vi "探头窗口-12-网络版.vi"() -> ()   [LabVIEW 2017]
panel:
  in  "外部停止命令？":bool=TRUE
  out "引用-监测模式？":refnum<vi>
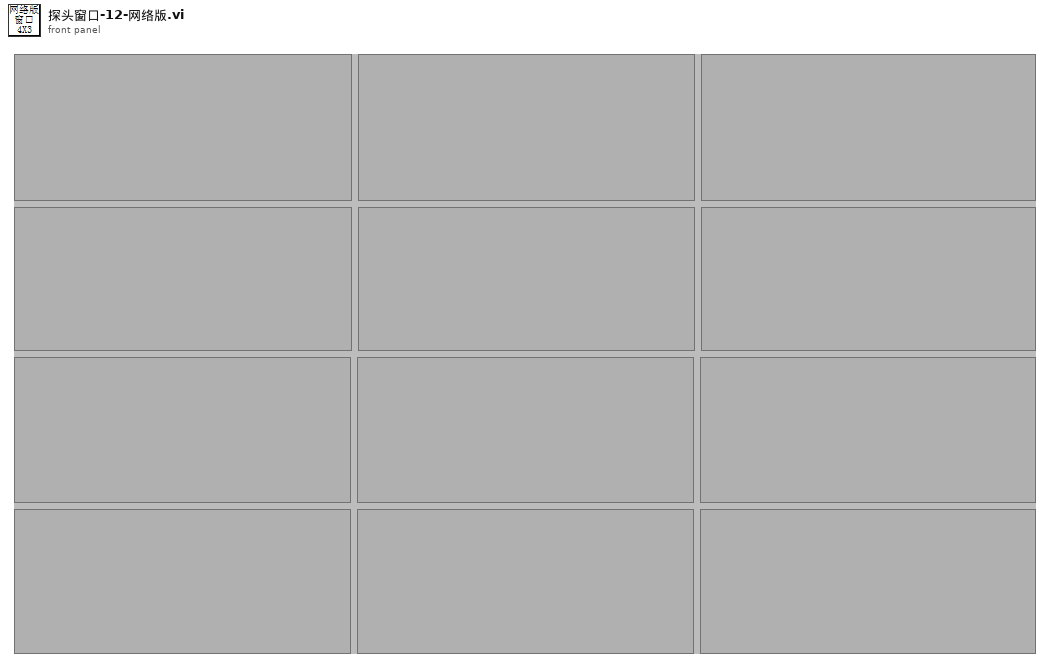
[diagram p1: front panel]
types:
  T1 = typedef "eventvkey.ctl" = enum16{"ASCII", "Enter", "Return", "Shift", "Ctrl", "Alt", "Cmd", "Opt", "Caps", "NumLock", "Clear", "Break", "Up", "Down", "Left", "Right", "Insert", "Delete", "Home", "End", "PageUp", "PageDown", "Escape", "Help", "Pause", "ScrollLock", "F1", "F2", "F3", "F4", "F5", "F6", "F7", "F8", "F9", "F10", "F11", "F12", "F13", "F14", "F15", "F16", "F17", "F18", "F19", "F20", "F21", "F22", "F23", "F24", "Play", "VolumeUp", "VolumeDown", "Mute", "Two Byte Char"}
  T2 = typedef "探头属性.ctl" = cluster{"探头地址与信息":T3, "测量值":T6, "限值":T7, "探头状态":T8, "累积记录":T9, "报警方式":T10}
  T3 = typedef "探测器信息.ctl" = cluster{"网络地址":string, "名称":string, "备注":string, "累积剂量":dbl, "累积限值":dbl, "硬件剂量率限值":T4, "剂量率限值1":dbl, "剂量率限值2":dbl, "报警方式":T5}
  T4 = typedef "探头剂量率限值选择.ctl" = enum16{"一级限值", "二级限值"}
  T5 = typedef "报警方式选择.ctl" = enum16{"常报警", "自动静音", "手动静音"}
  T6 = typedef "测量值.ctl" = cluster{"时间":timestamp, "数值":dbl}
  T7 = typedef "剂量率限值.ctl" = cluster{"限值1":dbl, "限值2":dbl, "探头限值":T4}
  T8 = typedef "探头状态.ctl" = enum16{"正常", "离线", "禁用", "一级报警", "二级报警", "累积报警"}
  T9 = typedef "单条累积记录.ctl" = cluster{"起始时间":timestamp, "结束时间":timestamp, "累积剂量":dbl}
  T10 = typedef "报警方式.ctl" = cluster{"报警方式":T5, "延迟计时":u16, "报警中？":bool}
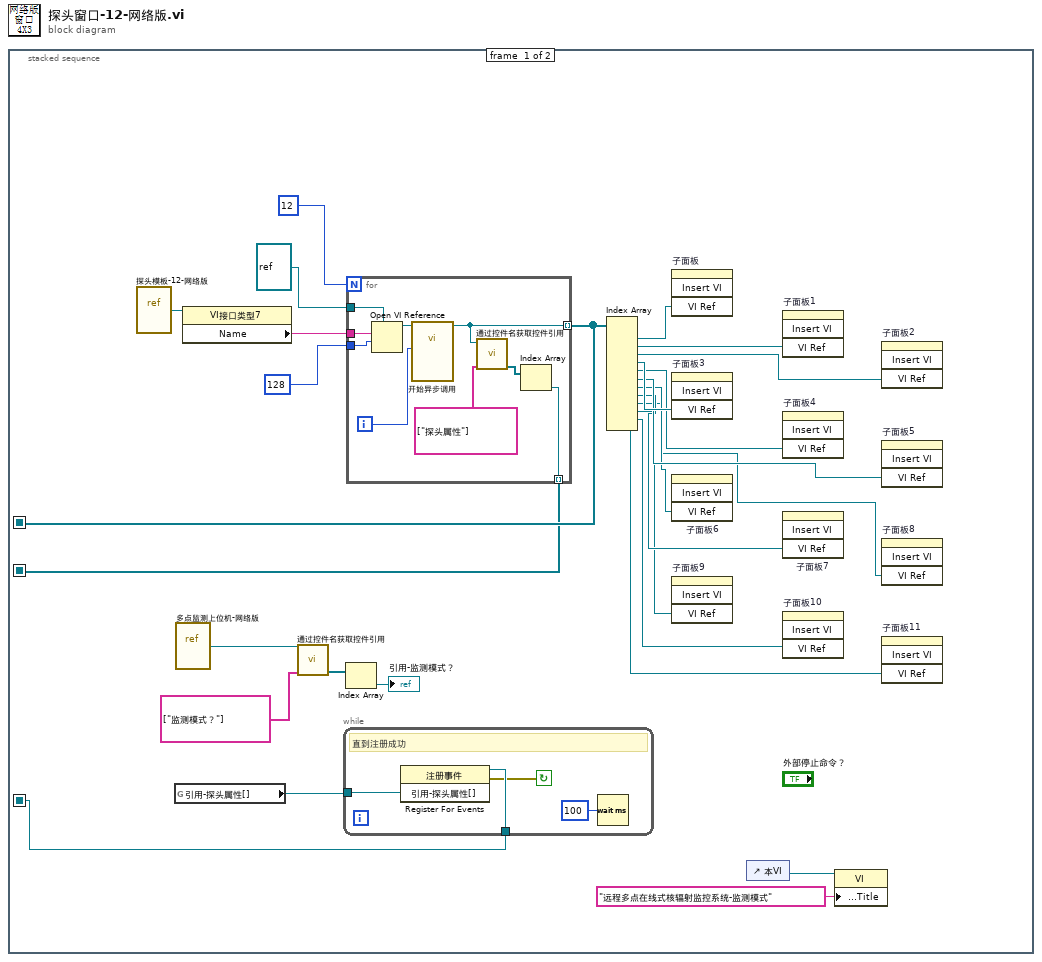
[diagram p0: block diagram]
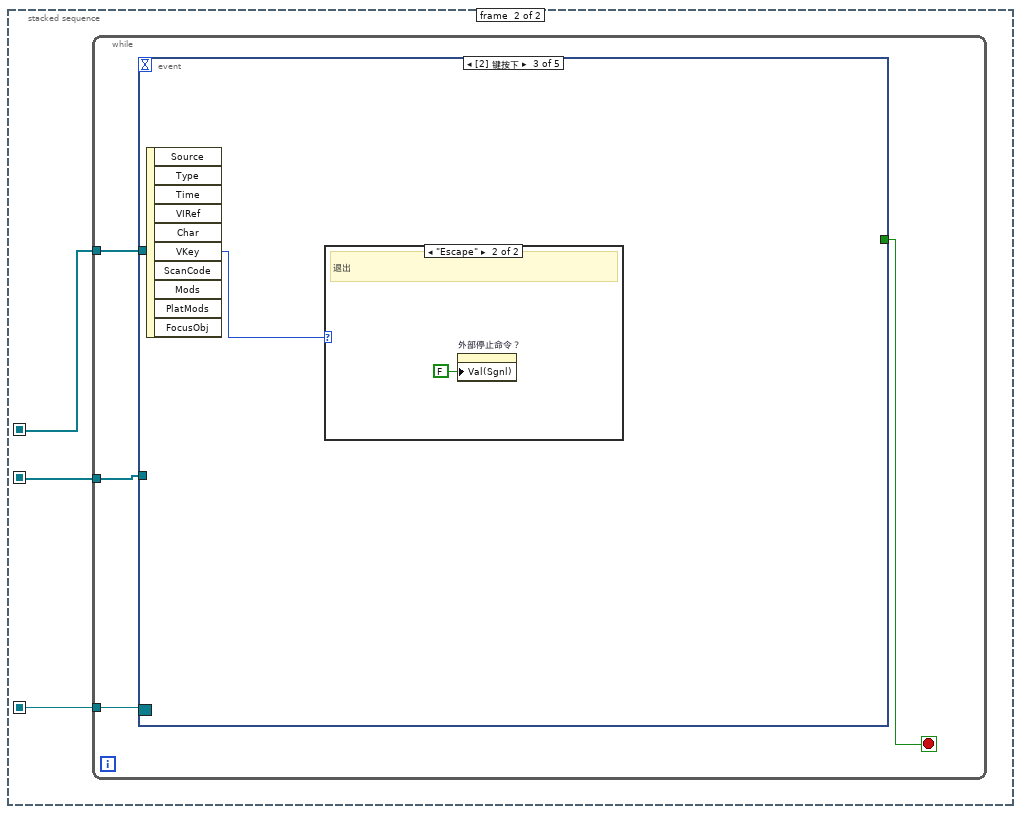
[diagram p2: hidden frame]
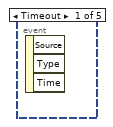
[diagram p3: hidden frame]
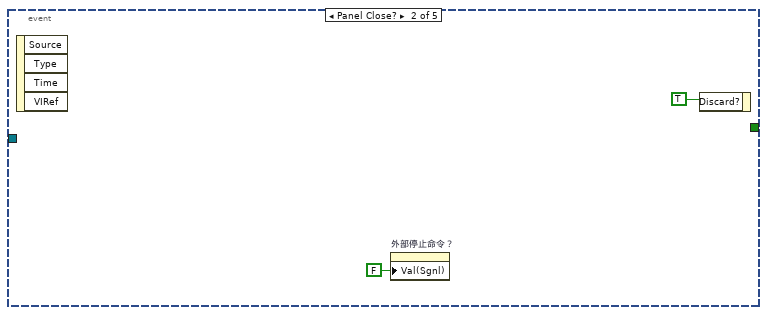
[diagram p4: hidden frame]
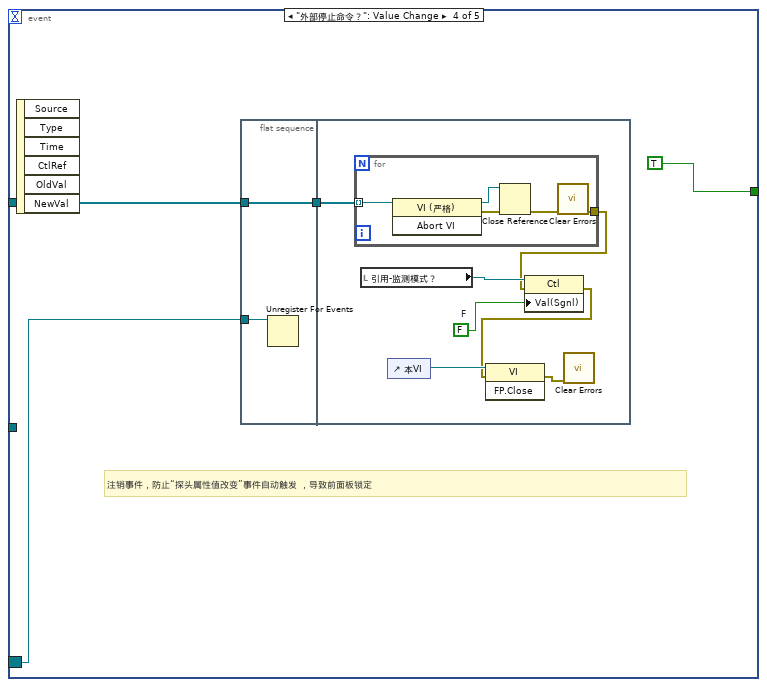
[diagram p6: hidden frame]
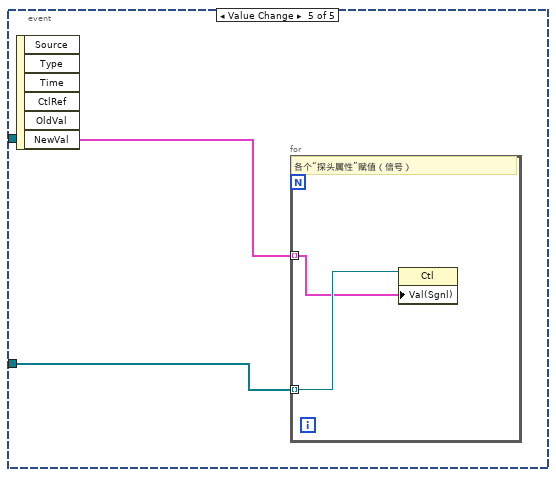
[diagram p7: hidden frame]
diagram:
  n1 = stacked-sequence {
    seq-local: [w23 _] -> [_ w43]
    seq-local: [w21 _] -> [_ w42]
    seq-local: [w1 _] -> [_ w41]
    frame #0 {
      n2 = vi-ref "探头模板-12-网络版.vi"() -> (w27:refnum<vi>)
      n3 = global read "全局变量-35点监测.vi" "引用-探头属性[]"() -> (w2:refnum<vi>)
      n4 = vi-ref "多点监测上位机-网络版.vi"() -> (w5:refnum<vi>)
      n5 = property class="VI接口类型7"(reference=w27) -> ("Name"=w26:string)  [unwired: 1 in, 2 out]
      n6 = call "通过控件名获取控件引用.vi"("控件名数组"=string[] ["监测模式？"], "VI引用"=w5) -> ("控件引用输出"=w7:refnum<vi>[])  [unwired: 7 in, 2 out]
      n7 = while {
        tunnel: w2 -> [w31]
        tunnel: [w30] -> w1
        stop <- w29 continue-if-true
        # "直到注册成功"
        n8 = register-events(w31) -> (reference out=w30:refnum<event-registration>, error out=w29:errorcluster)  [unwired: 2 in]
        n9 = Wait (ms)(milliseconds to wait=u32 100 ("等待时间（毫秒）")) -> ()  [unwired: 1 out]
      }
      n10 = Index Array(array=w7) -> (element=→"引用-监测模式？":refnum<vi>)  [unwired: 1 in]
      n11 = for "For循环" {
        N: 12 -> [_]
        tunnel: w26 -> [w40]
        tunnel: 128 ("选项") -> [w39]
        tunnel: refnum<vi> refnum ("类型说明符VI引用句柄（仅用于类型）") -> [w38]
        tunnel: [w33] -> w23 mode=indexing
        tunnel: [w34] -> w21 mode=indexing
        i -> [w32]
        n12 = Open VI Reference(type specifier VI Refnum (for type only)=w38, vi path=w40, options=w39) -> (vi reference=w35:refnum<vi>)  [unwired: 3 in, 1 out]
        n13 = call-by-ref "开始异步调用"(reference=w35, "探头序号"=w32) -> (reference out=w33:refnum<vi>)  [unwired: 12 in, 1 out]
        n14 = call "通过控件名获取控件引用.vi"("控件名数组"=string[] ["探头属性"], "VI引用"=w33) -> ("控件引用输出"=w37:refnum<vi>[])  [unwired: 7 in, 2 out]
        n15 = Index Array(array=w37) -> (element=w34:refnum<vi>)  [unwired: 1 in]
      }
      n16 = Index Array(array=w23) -> (element #1=w20:refnum<vi>, element #2=w19:refnum<vi>, element #3=w18:refnum<vi>, element #4=w17:refnum<vi>, element #5=w16:refnum<vi>, element #6=w15:refnum<vi>, element #7=w14:refnum<vi>, element #8=w13:refnum<vi>, element #9=w12:refnum<vi>, element #10=w11:refnum<vi>, element #11=w10:refnum<vi>, element #12=w9:refnum<vi>)  [unwired: 12 in]
      n17 = invoke on="子面板" class="子面板" method="Insert VI"("VI Ref"=w20) -> ()  [unwired: 3 in, 4 out]
      n18 = invoke on="子面板3" class="SubPnl" method="Insert VI"("VI Ref"=w17) -> ()  [unwired: 3 in, 4 out]
      n19 = invoke on="子面板6" class="SubPnl" method="Insert VI"("VI Ref"=w14) -> ()  [unwired: 3 in, 4 out]
      n20 = invoke on="子面板9" class="SubPnl" method="Insert VI"("VI Ref"=w11) -> ()  [unwired: 3 in, 4 out]
      n21 = control-ref of="本VI"() -> (w4:refnum<vi>)
      n22 = invoke on="子面板1" class="SubPnl" method="Insert VI"("VI Ref"=w19) -> ()  [unwired: 3 in, 4 out]
      n23 = invoke on="子面板4" class="SubPnl" method="Insert VI"("VI Ref"=w16) -> ()  [unwired: 3 in, 4 out]
      n24 = invoke on="子面板7" class="SubPnl" method="Insert VI"("VI Ref"=w13) -> ()  [unwired: 3 in, 4 out]
      n25 = invoke on="子面板10" class="SubPnl" method="Insert VI"("VI Ref"=w10) -> ()  [unwired: 3 in, 4 out]
      n26 = property class="VI"(reference=w4, "Front Panel.Title"="远程多点在线式核辐射监控系统-监测模式" ("前面板窗口:标题")) -> ()  [unwired: 1 in, 2 out]
      n27 = invoke on="子面板2" class="SubPnl" method="Insert VI"("VI Ref"=w18) -> ()  [unwired: 3 in, 4 out]
      n28 = invoke on="子面板5" class="SubPnl" method="Insert VI"("VI Ref"=w15) -> ()  [unwired: 3 in, 4 out]
      n29 = invoke on="子面板8" class="SubPnl" method="Insert VI"("VI Ref"=w12) -> ()  [unwired: 3 in, 4 out]
      n30 = invoke on="子面板11" class="SubPnl" method="Insert VI"("VI Ref"=w9) -> ()  [unwired: 3 in, 4 out]
    }
    frame #1 {
      n31 = while {
        tunnel: w43 -> [w46]
        tunnel: w42 -> [w45]
        tunnel: w41 -> [w44]
        stop <- w47 stop-if-true
        n32 = event shown="[2] 键按下" {
          selector: w44 -> [_ _ _ w52 _]
          dyn-events: _ -> [_ _ _ _ _]
          timeout: _ -> [_ _ _ _ _]
          tunnel: [_ _ _ TRUE ("放弃？") _] -> w47
          tunnel: w46 -> [_ _ _ w54 _]
          tunnel: w45 -> [_ _ _ _ w70]
          event Timeout {
            n33 = event-data() -> ()  [unwired: 1 in, 3 out]
          }
          event Panel Close? {
            n34 = event-data() -> ()  [unwired: 1 in, 4 out]
            n35 = property on="外部停止命令？" class="Bool (严格)"("Val(Sgnl)"=FALSE ("值(信号)")) -> ()  [unwired: 2 in, 2 out]
            n36 = event-data("Discard?"=TRUE ("放弃？")) -> ()  [unwired: 1 in, 1 out]
          }
          event Key Down {
            n37 = event-data() -> ("VKey"=w50:T1)  [unwired: 1 in, 9 out]
            n38 = case shown="\"Escape\"" w50 {
              frame "ASCII", Default {
              }
              frame "Escape" {
                # "退出"
                n39 = property on="外部停止命令？" class="Bool (严格)"("Val(Sgnl)"=FALSE ("值(信号)")) -> ()  [unwired: 2 in, 2 out]
              }
            }
          }
          event "外部停止命令？": Value Change {
            # "注销事件，防止“探头属性值改变”事件自动触发 ，导致前面板锁定"
            n40 = event-data() -> ()  [unwired: 1 in, 6 out]
            n41 = flat-sequence {
              tunnel: w54 -> [w57]
              tunnel: [w57] -> w53
              tunnel: w52 -> [w56]
              tunnel: w53 -> [w64]
              frame #0 {
                n42 = Unregister For Events(event registration refnum=w56) -> ()  [unwired: 1 in, 1 out]
              }
              frame #1 {
                w62 = FALSE  # F
                n43 = for "For循环" {
                  tunnel: w64 -> [w69] mode=indexing
                  tunnel: [w65] -> w60
                  n44 = invoke class="VI (严格)" method="Abort VI"(reference=w69) -> (reference out=w67:refnum<vi>, error out=w68:errorcluster)  [unwired: 2 in, 1 out]
                  n45 = Close Reference(reference=w67, error in (no error)=w68) -> (error out=w66:errorcluster)
                  n46 = call <vilib>:"Clear Errors.vi"("error in (no error)"=w66) -> ("error out"=w65:errorcluster)  [unwired: 5 in, 1 out]
                }
                n47 = local read "引用-监测模式？"() -> (w63:refnum<vi>)
                n48 = control-ref of="本VI"() -> (w61:refnum<vi>)
                n49 = property class="Ctl"(reference=w63, error in=w60, "Val(Sgnl)"=w62) -> (error out=w59:errorcluster)  [unwired: 1 out]
                n50 = invoke class="VI" method="FP.Close"(reference=w61, error in=w59) -> (error out=w58:errorcluster)  [unwired: 1 in, 2 out]
                n51 = call <vilib>:"Clear Errors.vi"("error in (no error)"=w58) -> ()  [unwired: 5 in, 2 out]
              }
            }
          }
          event Value Change {
            n52 = event-data() -> ("NewVal"=w71:T2[])  [unwired: 1 in, 5 out]
            n53 = for "For循环" {
              tunnel: w70 -> [w73] mode=indexing
              tunnel: w71 -> [w72] mode=indexing
              # "各个“探头属性”赋值（信号）"
              n54 = property class="Ctl"(reference=w73, "Val(Sgnl)"=w72) -> ()  [unwired: 1 in, 2 out]
            }
          }
        }
      }
    }
  }
